vi "Receive.vi"(8 "error in (no error)":errorcluster, 9 "timeout in ms (0)":i32, 11 "Communication in":refnum<class "Network.lvclass">) -> (0 "error out":errorcluster, 1 "Timeout?":bool, 2 "Packet Received":refnum<class "Packet.lvclass">, 3 "Communication out":refnum<class "Network.lvclass">)   [LabVIEW 2020, in "Communication Classes.lvlib" / "Network.lvclass"]
uses:
  Network.lvclass
  IP_Communication/IP_Communication.lvclass
  Packet/Packet.lvclass
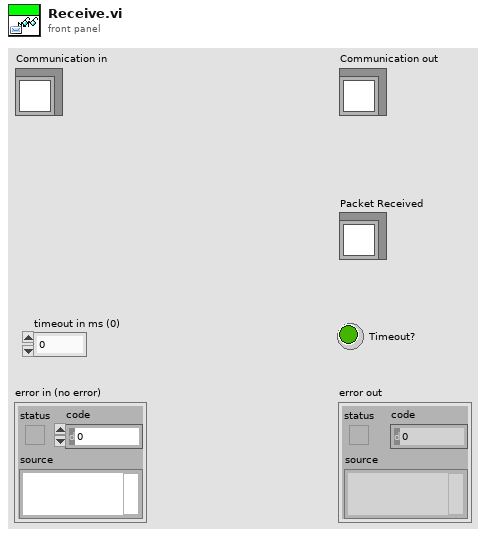
[diagram p1: front panel]
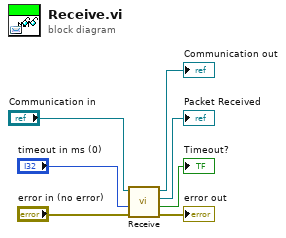
[diagram p0: block diagram]
diagram:
  n1 = call-parent "Receive.vi"("error in (no error)"="error in (no error)", "timeout in ms (0)"="timeout in ms (0)", "Communication in"="Communication in") -> ("error out"=→"error out":errorcluster, "Timeout?"=→"Timeout?":bool, "Packet Received"=→"Packet Received":refnum<class "Packet.lvclass">, "Communication out"=→"Communication out":refnum<class "Network.lvclass">)  [unwired: 5 in]
